vi "ForLoop_Double.vi"() -> ()   [LabVIEW 2018]
panel:
  out "x*y":i32[][](array[numeric])
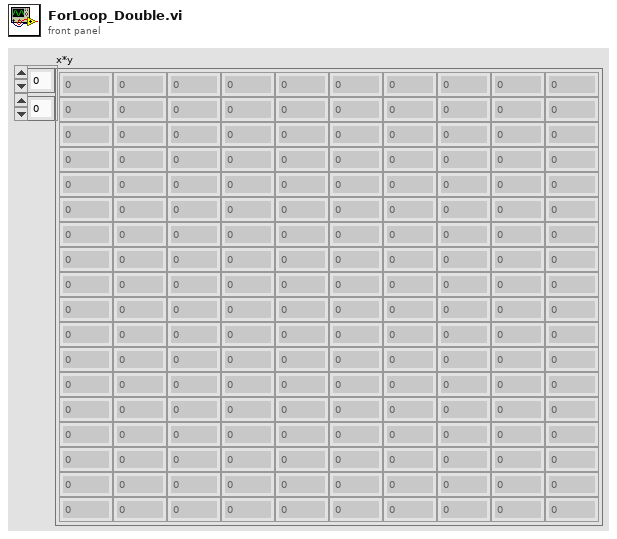
[diagram p1: front panel]
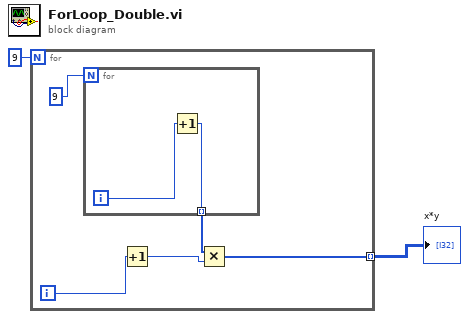
[diagram p0: block diagram]
diagram:
  n1 = for {
    N: 9 -> [_]
    tunnel: [w3] -> w1 mode=indexing
    i -> [w6]
    n2 = for {
      N: 9 -> [_]
      tunnel: [w8] -> w4 mode=indexing
      i -> [w9]
      n3 = Increment(x=w9) -> (x+1=w8:i32)
    }
    n4 = Increment(x=w6) -> (x+1=w5:i32)
    n5 = Multiply(x=w4, y=w5) -> (x*y=w3:i32[])
  }
  "x*y" <- w1
